vi "ReadyToKick.vi"(0 "object in":refnum<class "PrepareShootTactic.lvclass">, 5 "error in (no error)":errorcluster) -> (14 "object out":refnum<class "PrepareShootTactic.lvclass">, 16 "ready":bool=TRUE, 19 "error out":errorcluster)   [LabVIEW 2023, in "PrepareShootTactic.lvclass"]
uses:
  PrepareShootTactic.lvclass
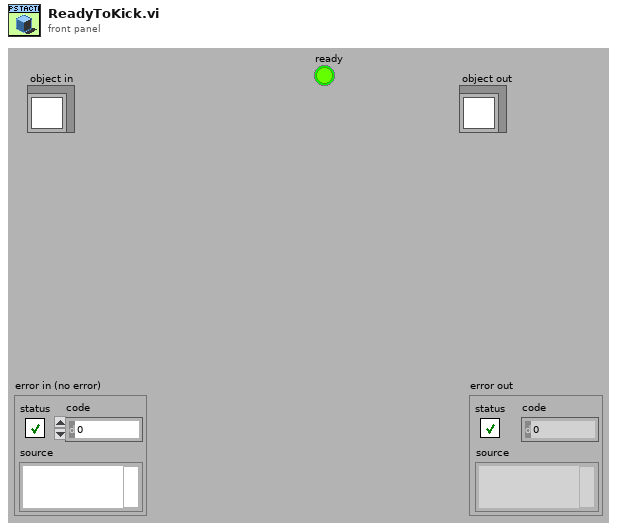
[diagram p1: front panel]
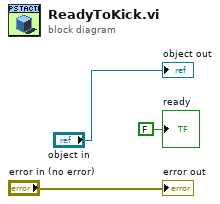
[diagram p0: block diagram]
diagram:
  "error out" <- "error in (no error)"
  "object out" <- "object in"
  "ready" <- FALSE ("ready")
